vi "Konvolucio MCAN120803 Example Tool.vi"() -> ()   [LabVIEW 2011]
uses:
  <vilib>/Utility/miscctls.llb/LVRowAndColumnUnsignedTypeDef.ctl
  <instrlib>/Konvolucio MCAN120803/Types/CanHandleType.ctl
  <vilib>/Utility/sysdir.llb/System Directory Type.ctl
  <instrlib>/Konvolucio MCAN120803/Types/MessageType.ctl
  <instrlib>/Konvolucio MCAN120803/Public/Attributes/AttrGetRxPendingMsg.vi
  <instrlib>/Konvolucio MCAN120803/Public/Attributes/AttrGetTxPendingMsg.vi
  <instrlib>/Konvolucio MCAN120803/Public/Attributes/AttrGetRxTotal.vi
  <instrlib>/Konvolucio MCAN120803/Public/Attributes/AttrGetTxTotal.vi
  <instrlib>/Konvolucio MCAN120803/Public/Attributes/AttrGetRxErrorCounter.vi
  <instrlib>/Konvolucio MCAN120803/Public/Attributes/AttrGetTxErrorCounter.vi
  <instrlib>/Konvolucio MCAN120803/Public/Attributes/AttrGetRxDrop.vi
  <instrlib>/Konvolucio MCAN120803/Public/Attributes/AttrGetTxDrop.vi
  <instrlib>/Konvolucio MCAN120803/Public/Attributes/AttrSetLoopback.vi
  <instrlib>/Konvolucio MCAN120803/Public/Attributes/AttrSetListenOnly.vi
  <instrlib>/Konvolucio MCAN120803/Public/Attributes/AttrGetAssemblyVersion.vi
  <instrlib>/Konvolucio MCAN120803/Public/Attributes/AttrSetNonAutoRetransmission.vi
  <instrlib>/Konvolucio MCAN120803/Public/Attributes/AttrGetFirmwareRev.vi
  <instrlib>/Konvolucio MCAN120803/Public/Attributes/AttrGetSerialNumber.vi
  <instrlib>/Konvolucio MCAN120803/Public/Attributes/AttrSetTermination.vi
  C:/Program Files/National Instruments/LabVIEW 2011/instr.lib/Konvolucio MCAN120803/Private/Konvolucio.MCAN120803.API.dll
  Private/Konvolucio.MCAN120803.API.dll
  <instrlib>/Konvolucio MCAN120803/Konvolucio MCAN120803.lvlib
panel:
  out "ledStop":bool
  in  "checkBoxListenOnly":bool
  in  "checkBoxNoAutoTx":bool
  in  "checkBoxTermination":bool
  in  "checkBoxLoopback":bool
  in  "Tab 4":enum32{"Incoming messages"}(tab)
  in  "buttonAutoScroll":bool
  in  "buttonSave":bool
  out "Table Control":string[][](table)
  in  "buttonClear":bool
  out "TableRecords":i32
  in  "Tab 3":enum32{"Adapter Info"}(tab)
  out "Serial Number":string
  out "Fw Revision":string
  out "Asm Version":string
  in  "Tab 2":enum32{"Diag"}(tab)
  out "Tx Pending":u32
  out "Rx Pending":u32
  out "Tx Drop":u32
  out "Rx Drop":u32
  out "Tx Error":u32
  out "Rx Error":u32
  out "Tx Total":u32
  out "Rx Total":u32
  in  "Tab":enum32{"Send Simple Message "}(tab)
  in  "buttonSendC":bool
  in  "dataFrameC":string
  in  "lengthC":u8 format="%02x"
  in  "arbIdC":u32 format="%08x"
  in  "buttonSendB":bool
  in  "dataFrameB":string
  in  "lengthB":u8 format="%02x"
  in  "arbIdB":u32 format="%08x"
  in  "dataFrameA":string
  in  "lengthA":u8 format="%02x"
  in  "arbIdA":u32 format="%08x"
  in  "buttonSendA":bool
  in  "comboBaudRate":i32(ring) items=["5.000kBaud", "5.555kBaud", "6.250kBaud", "8.000kBaud", "10.000kBaud", "12.500kBaud", "15.625kBaud", "16.000kBaud", "20.000kBaud", "25.000kBaud", "31.250kBaud", "33.333kBaud", "40.000kBaud", "50.000kBaud", "62.250kBaud", "80.000kBaud", "83.333kBaud", "100.000kBaud", "125.000kBaud", "166.666kBaud", "200.000kBaud", "250.000kBaud", "400.000kBaud", "500.000kBaud", "800.000kBaud", "1.000MBaud"]
  in  "buttonPause":bool
  out "ledOpen":bool
  in  "buttonPlay":bool
  in  "buttonStop":bool
  in  "comboAdapters":i32(ring) items=["CAN Bus Adpater - MCAN120803 3873366E3133 "]
  # "Adapter:"
  # "A"
  # "B"
  # "C"
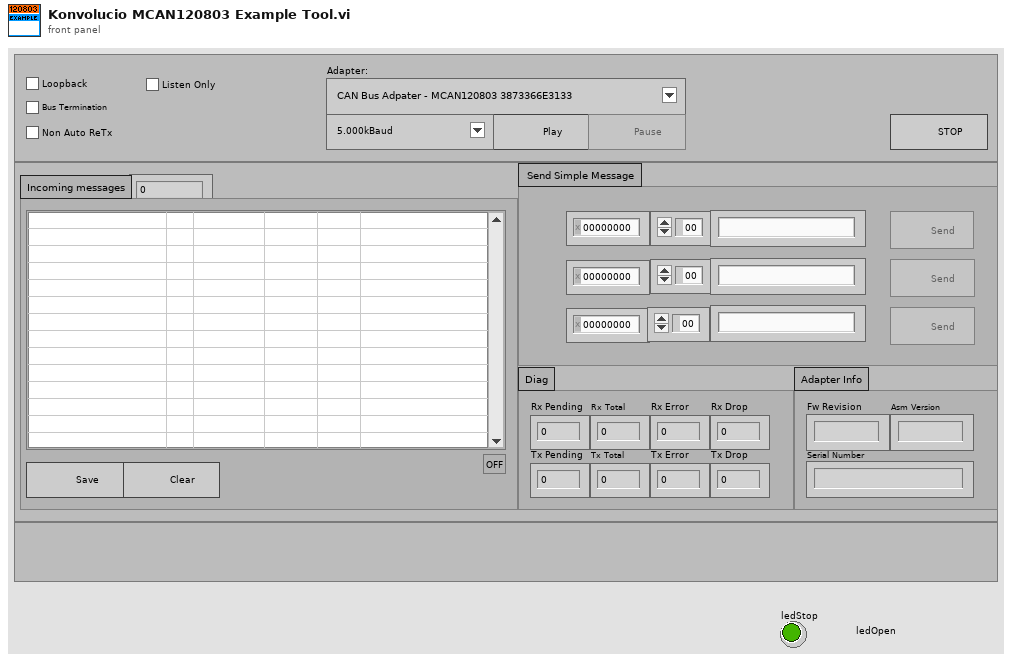
[diagram p1: front panel]
types:
  T1 = enum8{"Enabled", "Disabled", "Disabled and Grayed Out"}
  T2 = typedef "LVRowAndColumnUnsignedTypeDef.ctl" = cluster{"Row":u32, "Column":u32}
  T3 = typedef "Konvolucio MCAN120803.lvlib/BaudRateItemType.ctl" = cluster{"Name":string, "Value":u32}
  T4 = typedef "Konvolucio MCAN120803.lvlib/AdapterItemType.ctl" = cluster{"Name":string, "DeviceDescription":string, "SerialNumber":string, "InUse":bool, "Handle":refnum<k24>}
  T5 = typedef "Konvolucio MCAN120803.lvlib/CanHandleType.ctl" = cluster{"AdapterDevice":refnum<k24>}
  T6 = enum16{"open", "replace", "create", "open or create", "replace or create", "replace or create with confirmation"}
  T7 = typedef "Konvolucio MCAN120803.lvlib/MessageType.ctl" = cluster{"TimeStamp":timestamp, "ArbitrationId":u32, "IsRemote":u8, "DataLength":u8, "Data":u8[]}
  T8 = typedef "System Directory Type.ctl" = i32
  T9 = cluster{"Shift":bool, "Ctrl":bool, "Alt":bool, "Cmd":bool, "Opt":bool}
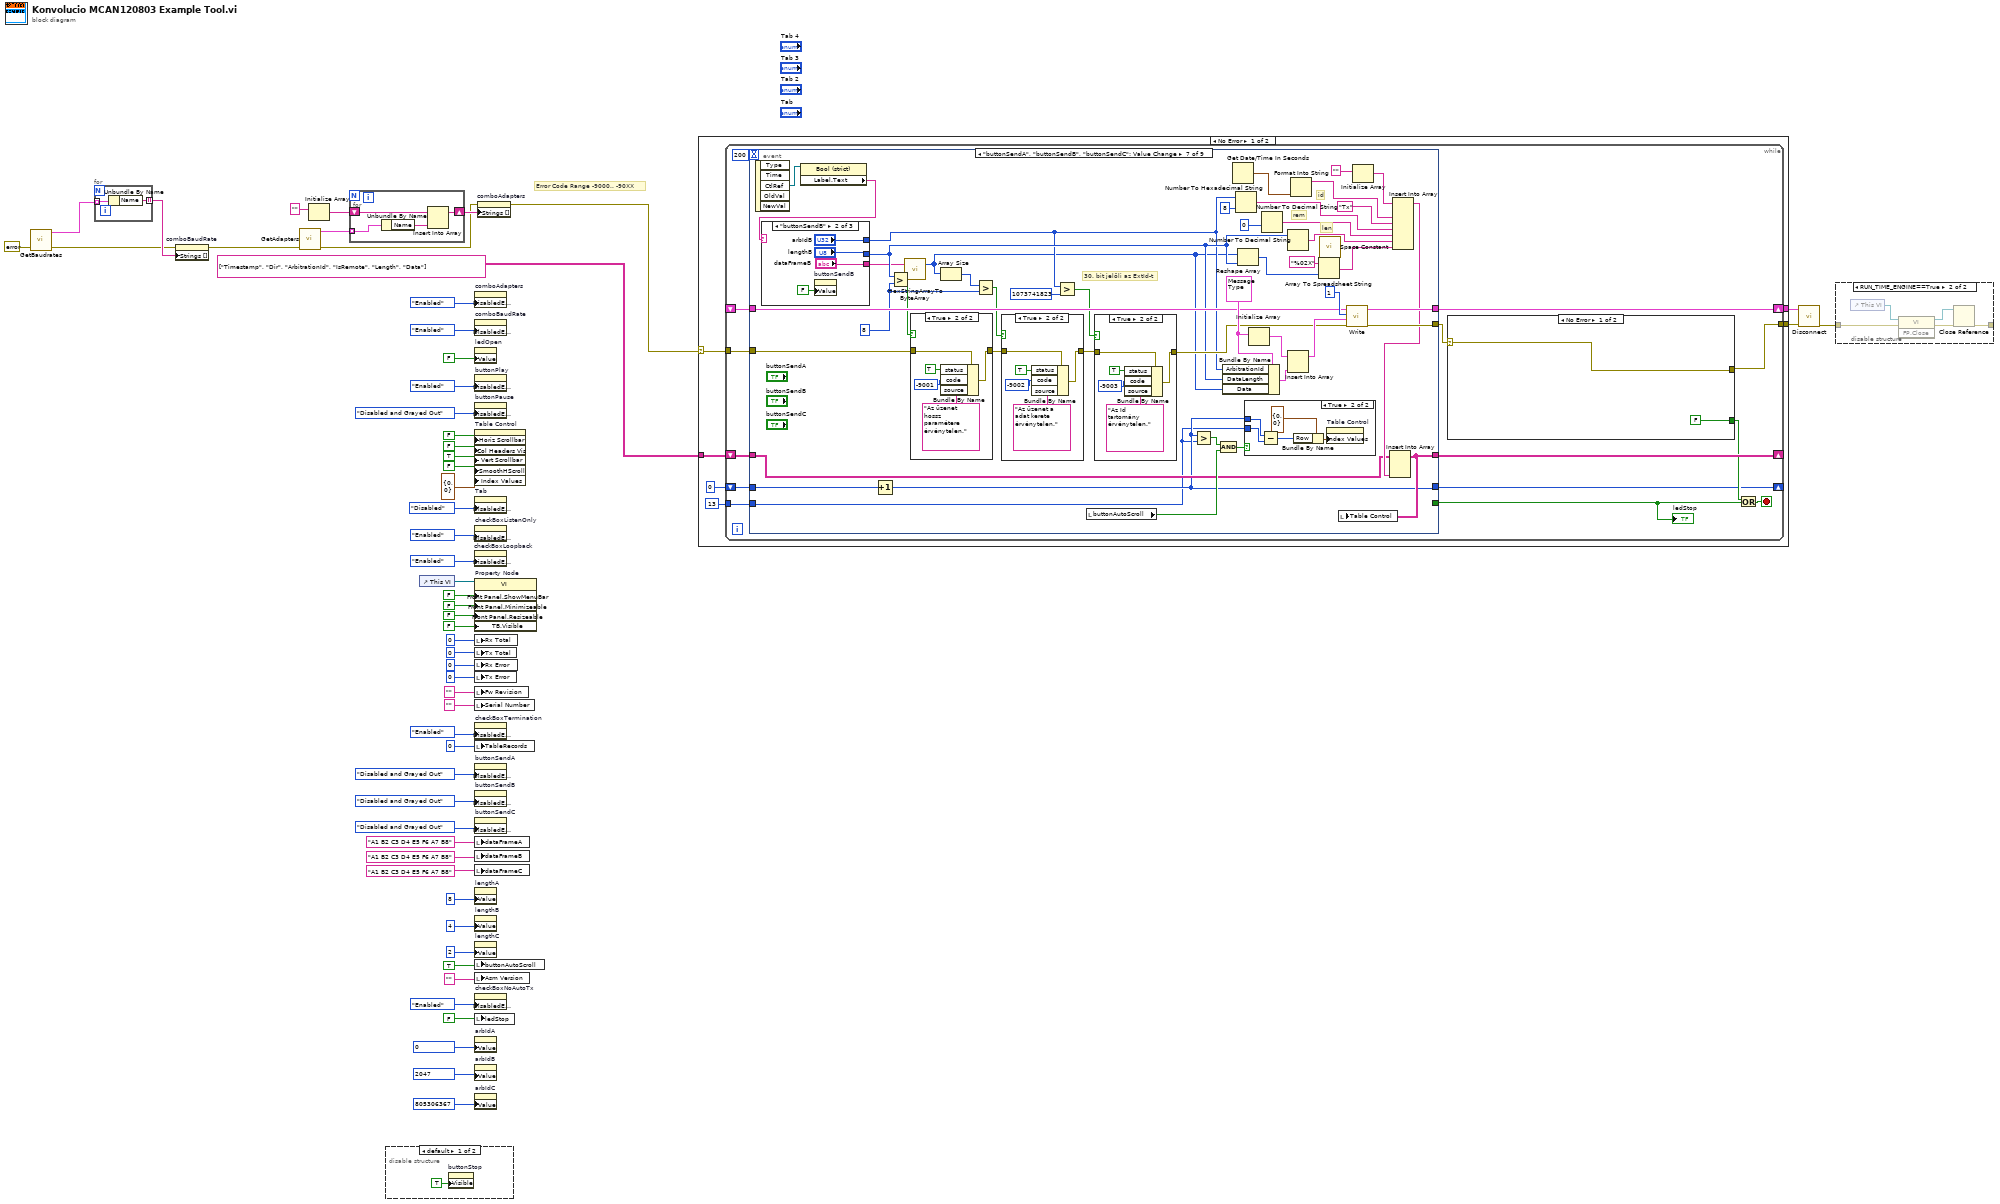
[diagram p0: block diagram]
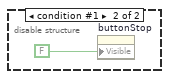
[diagram p2: hidden frame]
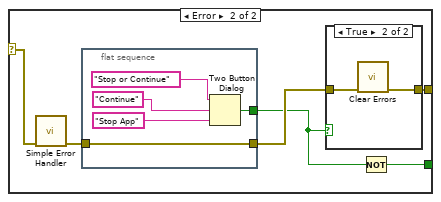
[diagram p4: hidden frame]
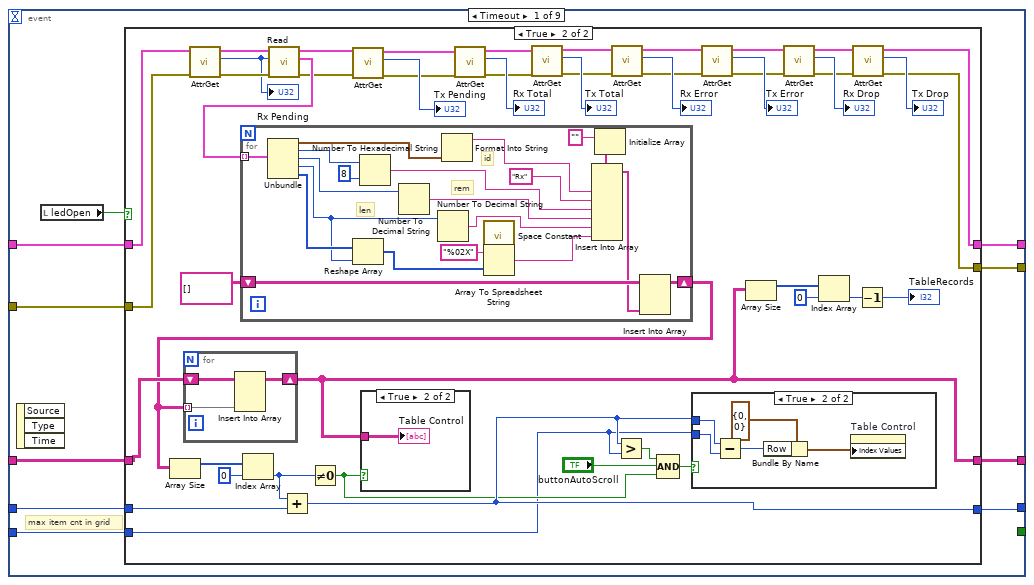
[diagram p6: hidden frame]
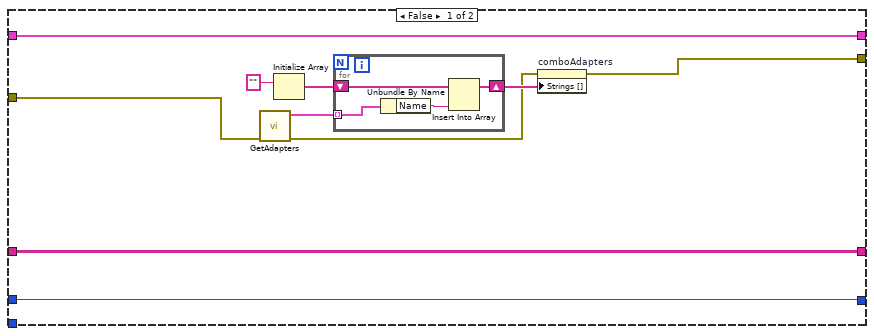
[diagram p7: hidden frame]
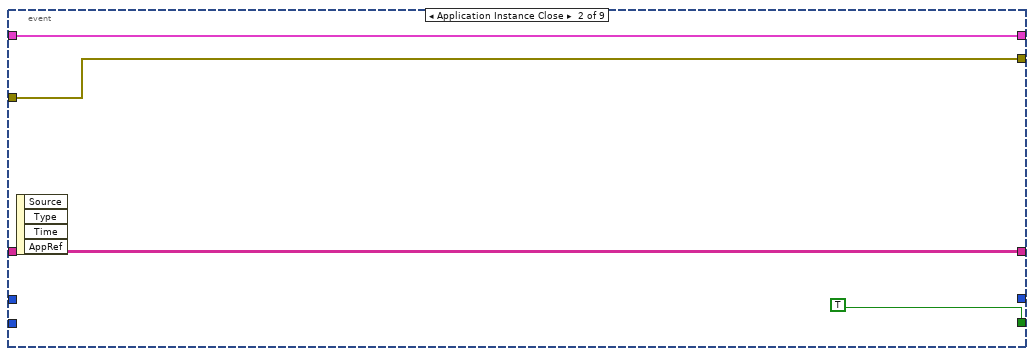
[diagram p10: hidden frame]
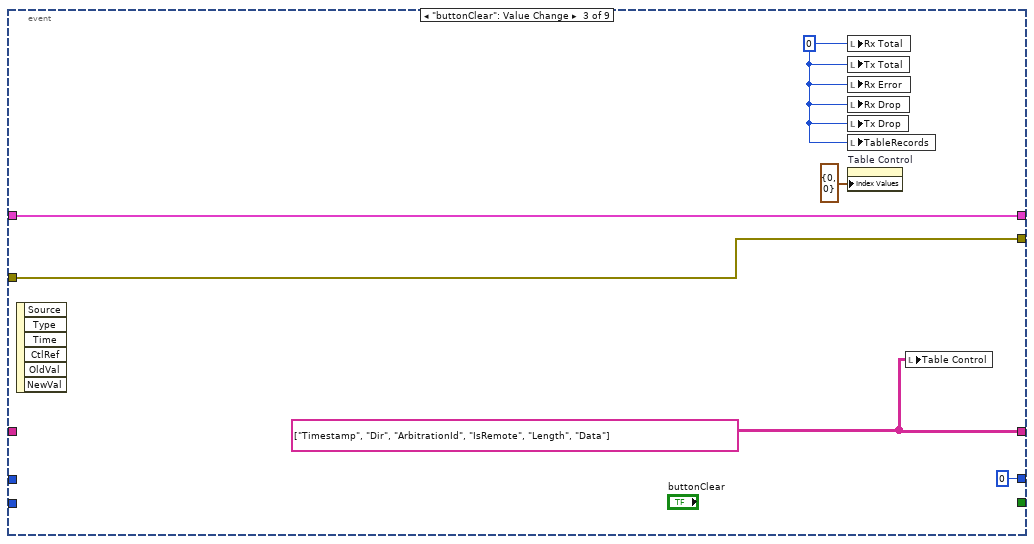
[diagram p11: hidden frame]
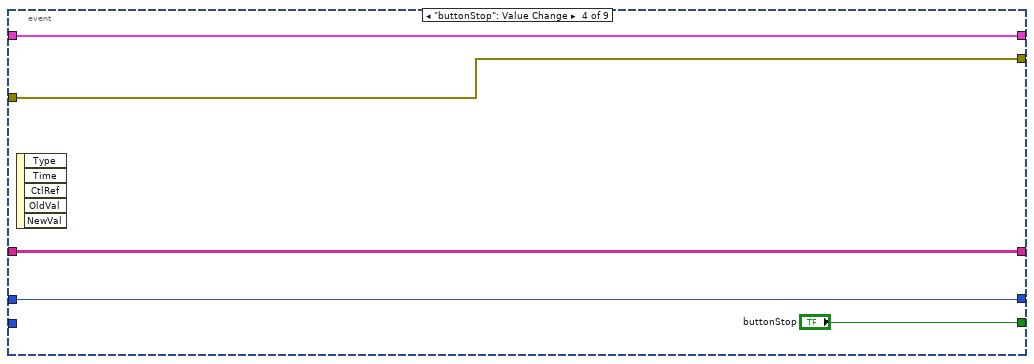
[diagram p12: hidden frame]
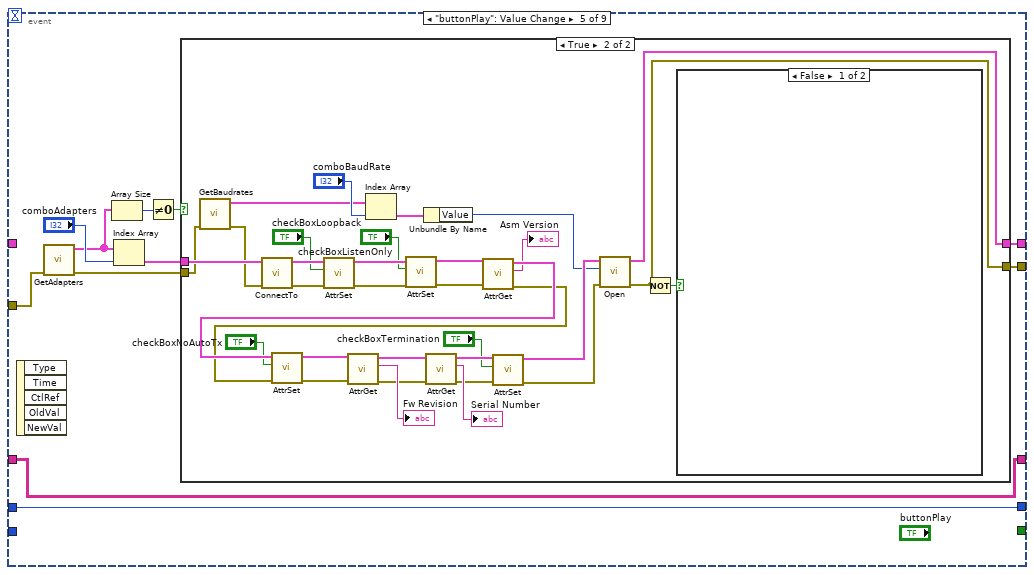
[diagram p13: hidden frame]
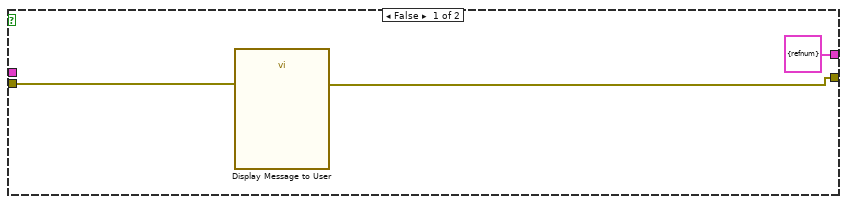
[diagram p14: hidden frame]
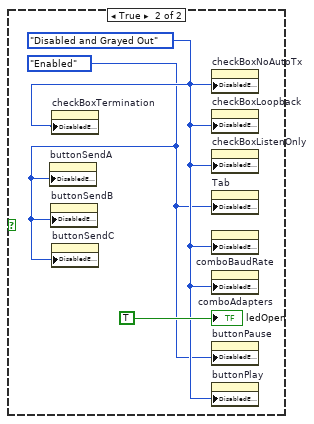
[diagram p15: hidden frame]
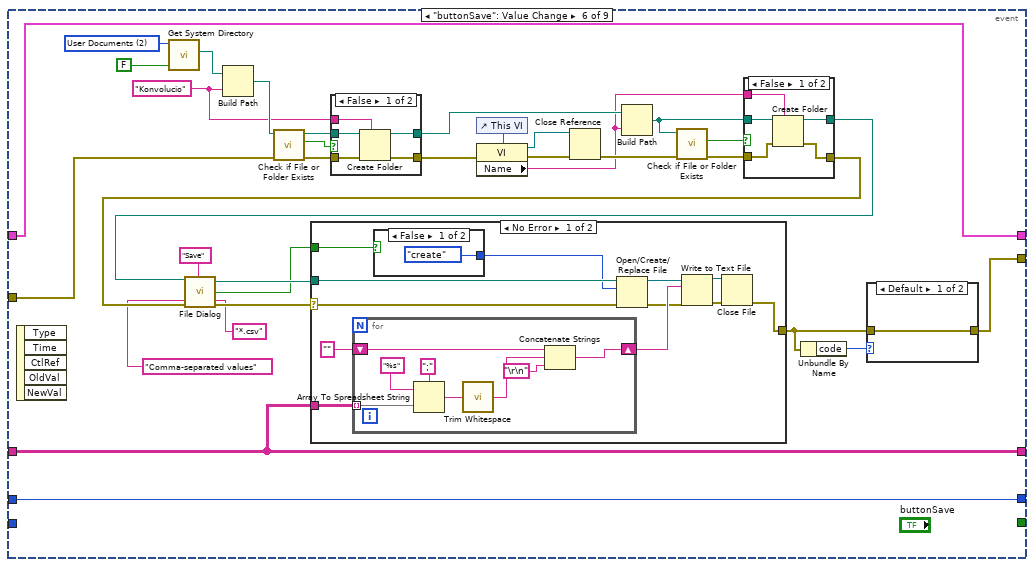
[diagram p16: hidden frame]
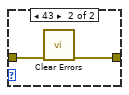
[diagram p17: hidden frame]
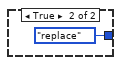
[diagram p18: hidden frame]
diagram:
  # "Error Code Range -9000.. -90XX"
  n1 = call <instrlib>:"GetBaudrates.vi"("error in"=errorcluster {"status"=FALSE, "code"=0, "source"=""}) -> ("error out"=w21:errorcluster, "BaudRateCollection"=w22:T3[])  [unwired: 9 in]
  n2 = for {
    tunnel: w22 -> [w59] mode=indexing
    tunnel: [w58] -> w46 mode=indexing
    n3 = Unbundle By Name(w59) -> ("Name"=w58:string)
  }
  n4 = property on="comboBaudRate" class="Ring (strict)"(error in=w21, "Strings []"=w46) -> (error out=w20:errorcluster)  [unwired: 1 in, 1 out]
  n5 = call <instrlib>:"GetAdapters.vi"("error in"=w20) -> ("error out"=w48:errorcluster, "AdaptersOut"=w57:T4[])  [unwired: 9 in]
  n6 = Initialize Array("") -> (w49:string[])  [unwired: 1 in]
  n7 = for {
    tunnel: w57 -> [w61] mode=indexing
    shift-right: [w62] -> w55
    shift-left: w49 -> [w60]
    n8 = Unbundle By Name(w61) -> ("Name"=w63:string)
    n9 = Insert Into Array(array=w60, new element=w63) -> (w62:string[])  [unwired: 1 in]
  }
  n10 = disable-structure shown="default" {
    frame condition #0 (active) {
      n11 = property on="buttonStop" class="Bool"("Visible"=TRUE) -> ()  [unwired: 2 in, 2 out]
    }
    frame condition #1 {
      n12 = property on="buttonStop" class="Bool"("Visible"=FALSE) -> ()  [unwired: 2 in, 2 out]
    }
  }
  n13 = control-ref of="This VI"() -> (w38:refnum<vi>)
  n14 = property on="comboAdapters" class="Ring (strict)"("DisabledEnum"=T1."Enabled" ("Disabled")) -> ()  [unwired: 2 in, 2 out]
  n15 = property on="comboBaudRate" class="Ring (strict)"("DisabledEnum"=T1."Enabled" ("Disabled")) -> ()  [unwired: 2 in, 2 out]
  n16 = property on="ledOpen" class="Bool (strict)"("Value"=FALSE ("Open")) -> ()  [unwired: 2 in, 2 out]
  n17 = property on="buttonPlay" class="Bool"("DisabledEnum"=T1."Enabled" ("Disabled")) -> ()  [unwired: 2 in, 2 out]
  n18 = property on="buttonPause" class="Bool"("DisabledEnum"=T1."Disabled and Grayed Out" ("Disabled")) -> ()  [unwired: 2 in, 2 out]
  n19 = property on="Table Control" class="Tbl (strict)"("Horiz Scrollbar"=FALSE ("Visible Items:Vertical Scrollbar Visible"), "Col Headers Vis"=FALSE ("Visible Items:Column Headers Visible"), "Vert Scrollbar"=TRUE ("Visible Items:Vertical Scrollbar Visible"), "SmoothHScroll"=FALSE ("Smooth Horizontal Scrolling"), "Index Values"=T2 {"Row"=0, "Column"=0}) -> ()  [unwired: 2 in, 2 out]
  n20 = property on="Tab" class="TabCtl (strict)"("DisabledEnum"=T1."Disabled" ("Disabled")) -> ()  [unwired: 2 in, 2 out]
  n21 = property on="checkBoxListenOnly" class="Bool (strict)"("DisabledEnum"=T1."Enabled" ("Disabled")) -> ()  [unwired: 2 in, 2 out]
  n22 = property on="checkBoxLoopback" class="Bool (strict)"("DisabledEnum"=T1."Enabled" ("Disabled")) -> ()  [unwired: 2 in, 2 out]
  n23 = property on="Property Node" class="VI"(reference=w38, "Front Panel.ShowMenuBar"=FALSE ("Front Panel Window:Show Menu Bar"), "Front Panel.Minimizeable"=FALSE ("Front Panel Window:Minimizable"), "Front Panel.Resizeable"=FALSE ("Front Panel Window:Resizable"), "TB.Visible"=FALSE ("Tool Bar:Visible")) -> ()  [unwired: 1 in, 2 out]
  n24 = local write "Rx Total"(u32 0 ("Total Rx")) -> ()
  n25 = local write "Tx Total"(u32 0 ("Total Tx")) -> ()
  n26 = local write "Rx Error"(u32 0 ("Rx Error Counter")) -> ()
  n27 = local write "Tx Error"(u32 0 ("Tx Error Counter")) -> ()
  n28 = local write "Fw Revision"("" ("Firmware Revision")) -> ()
  n29 = local write "Serial Number"("" ("Serial Number")) -> ()
  n30 = property on="checkBoxTermination" class="Bool (strict)"("DisabledEnum"=T1."Enabled" ("Disabled")) -> ()  [unwired: 2 in, 2 out]
  n31 = local write "TableRecords"(u32 0 ("TableRecords")) -> ()
  n32 = property on="buttonSendA" class="Bool (strict)"("DisabledEnum"=T1."Disabled and Grayed Out" ("Disabled")) -> ()  [unwired: 2 in, 2 out]
  n33 = property on="buttonSendB" class="Bool (strict)"("DisabledEnum"=T1."Disabled and Grayed Out" ("Disabled")) -> ()  [unwired: 2 in, 2 out]
  n34 = property on="buttonSendC" class="Bool (strict)"("DisabledEnum"=T1."Disabled and Grayed Out" ("Disabled")) -> ()  [unwired: 2 in, 2 out]
  n35 = local write "dataFrameA"("A1 B2 C3 D4 E5 F6 A7 B8" ("dataFrame1")) -> ()
  n36 = local write "dataFrameB"("A1 B2 C3 D4 E5 F6 A7 B8" ("dataFrameB")) -> ()
  n37 = local write "dataFrameC"("A1 B2 C3 D4 E5 F6 A7 B8" ("dataFrameB")) -> ()
  n38 = property on="lengthA" class="DigNum (strict)"("Value"=u8 8 ("lengthA")) -> ()  [unwired: 2 in, 2 out]
  n39 = property on="lengthB" class="DigNum (strict)"("Value"=u8 4 ("lengthB")) -> ()  [unwired: 2 in, 2 out]
  n40 = property on="lengthC" class="DigNum (strict)"("Value"=u8 2 ("lengthC")) -> ()  [unwired: 2 in, 2 out]
  n41 = local write "buttonAutoScroll"(TRUE ("buttonAutoScroll")) -> ()
  n42 = local write "Asm Version"("" ("Asm Version")) -> ()
  n43 = property on="checkBoxNoAutoTx" class="Bool (strict)"("DisabledEnum"=T1."Enabled" ("Disabled")) -> ()  [unwired: 2 in, 2 out]
  n44 = local write "ledStop"(FALSE ("ledStop")) -> ()
  n45 = property on="arbIdA" class="DigNum (strict)"("Value"=u32 0 ("arbIdA")) -> ()  [unwired: 2 in, 2 out]
  n46 = property on="arbIdB" class="DigNum (strict)"("Value"=u32 2047 ("arbIdA")) -> ()  [unwired: 2 in, 2 out]
  n47 = property on="arbIdC" class="DigNum (strict)"("Value"=u32 805306367 ("arbIdA")) -> ()  [unwired: 2 in, 2 out]
  n48 = property on="comboAdapters" class="Ring (strict)"(error in=w48, "Strings []"=w55) -> (error out=w47:errorcluster)  [unwired: 1 in, 1 out]
  n49 = case shown="No Error" w47 {
    selector: w47 -> [w71 w450]
    tunnel: [w70 w450] -> w19
    tunnel: [w69 T5 {"AdapterDevice"=refnum} ("HandleOut")] -> w54
    tunnel: string[][] [["Timestamp", "Dir", "ArbitrationId", "IsRemote", "Length", "Data"]] ("Table Control 3") -> [w68 _]
    frame No Error {
      n50 = while {
        tunnel: w71 -> [w85]
        tunnel: [w75] -> w70
        shift-right: [w84] -> w69
        shift-left: _ -> [w83]
        shift-right: [w80] -> _
        shift-left: w68 -> [w81]
        shift-right: [w74] -> _
        shift-left: 0 ("x-1") -> [w73]
        tunnel: 13 ("y") -> [w72]
        stop <- w79 stop-if-true
        n51 = event shown="[6] \"buttonSendA\", \"buttonSendB\", \"buttonSendC\": Value Change" {
          selector: _ -> [_ _ _ _ _ _ _ _ _]
          dyn-events: _ -> [_ _ _ _ _ _ _ _ _]
          timeout: 200 -> [_ _ _ _ _ _ _ _ _]
          tunnel: [_ TRUE ("buttonStop") _ "buttonStop" _ _ _ _ _] -> w76
          tunnel: w85 -> [w110 w204 w211 w214 w223 w286 w359 w428 w446]
          tunnel: [w109 w204 w211 w214 w225 w269 w383 w428 w447] -> w78
          tunnel: [w108 w205 w212 w216 w226 w272 w381 w427 w444] -> w84
          tunnel: w83 -> [w111 w205 w212 w216 _ w272 w380 w427 w444]
          tunnel: w81 -> [w107 w203 _ w215 w218 w280 w358 w430 w437]
          tunnel: [w105 w203 w209 w215 w218 w280 w360 w430 w437] -> w80
          tunnel: [w103 _ 0 ("Total Rx") w213 w219 w268 w353 w429 w440] -> w74
          tunnel: w73 -> [w104 _ _ w213 w219 w268 w364 w429 w440]
          tunnel: w72 -> [w102 _ _ _ _ _ w352 _ _]
          event Timeout {
            # "max item cnt in grid"
            n52 = event-data() -> ()  [unwired: 1 in, 3 out]
            n53 = local read "ledOpen"() -> (w106:bool)
            n54 = case shown="True" w106 {
              tunnel: w111 -> [w121 w169]
              tunnel: w110 -> [w115 w170]
              tunnel: [w113 w150] -> w109
              tunnel: [w121 w149] -> w108
              tunnel: w107 -> [w120 w143]
              tunnel: [w120 w144] -> w105
              tunnel: w104 -> [w112 w140]
              tunnel: [w112 w139] -> w103
              tunnel: w102 -> [_ w132]
              frame False {
                n55 = call <instrlib>:"GetAdapters.vi"("error in"=w115) -> ("error out"=w114:errorcluster, "AdaptersOut"=w116:T4[])  [unwired: 9 in]
                n56 = Initialize Array("") -> (w118:string[])  [unwired: 1 in]
                n57 = for {
                  tunnel: w116 -> [w123] mode=indexing
                  shift-right: [w124] -> w119
                  shift-left: w118 -> [w122]
                  n58 = Unbundle By Name(w123) -> ("Name"=w125:string)
                  n59 = Insert Into Array(array=w122, new element=w125) -> (w124:string[])  [unwired: 1 in]
                }
                n60 = property on="comboAdapters" class="Ring (strict)"(error in=w114, "Strings []"=w119) -> (error out=w113:errorcluster)  [unwired: 1 in, 1 out]
              }
              frame True {
                n61 = call-poly <instrlib>:"AttrGet.vi"("error in"=w170, "CanHandleIn"=w169) -> ("error out"=w171:errorcluster, "Value"=w131:i32, "CanHandleOut"=w172:T5)  [unwired: 7 in]
                "Rx Pending" <- w131
                n62 = call <instrlib>:"Read.vi"("error in"=w171, "Request Number of Message"=w131, "CanHandleIn"=w172) -> ("error out"=w130:errorcluster, "Messages"=w167:T7[], "CanHandleOut"=w129:T5)  [unwired: 6 in]
                n63 = for {
                  tunnel: w167 -> [w199] mode=indexing
                  shift-right: [w189] -> w138
                  shift-left: string[][] [] -> [w190]
                  # "len"
                  # "rem"
                  # "id"
                  n64 = Unbundle(w199) -> ("TimeStamp"=w187:timestamp, "ArbitrationId"=w194:u32, "IsRemote"=w195:u8, "DataLength"=w185:u8, "Data"=w196:u8[])
                  n65 = Reshape Array(w196, w185) -> (w186:u8[])
                  n66 = Number To Hexadecimal String(1:i16 8 ("width (-)"), 2:w194) -> (0:w181:string)
                  n67 = Number To Decimal String(number=w195) -> (decimal integer string=w182:string)  [unwired: 1 in]
                  n68 = Number To Decimal String(number=w185) -> (decimal integer string=w183:string)  [unwired: 1 in]
                  n69 = Format Into String(w187) -> (resulting string=w180:string)  [unwired: 3 in, 1 out]
                  n70 = call <vilib>:"Space Constant.vi"() -> ("String"=w197:string)
                  n71 = Array To Spreadsheet String(delimiter (Tab)=w197, array=w186, 3:"%02X" ("format string")) -> (spreadsheet string=w184:string)
                  n72 = Initialize Array("") -> (w192:string[])  [unwired: 1 in]
                  n73 = Insert Into Array(array=w192, new element #1=w180, new element #2="Rx" ("new element/subarray"), new element #3=w181, new element #4=w182, new element #5=w183, new element #6=w184) -> (w188:string[])  [unwired: 1 in]
                  n74 = Insert Into Array(array=w190, new element=w188) -> (w189:string[][])  [unwired: 2 in]
                }
                n75 = Array Size(array=w138) -> (size(s)=w142:i32[])
                n76 = for {
                  shift-right: [w202] -> w144
                  shift-left: w143 -> [w201]
                  tunnel: w138 -> [w200] mode=indexing
                  n77 = Insert Into Array(array=w201, new element=w200) -> (w202:string[][])  [unwired: 2 in]
                }
                n78 = Index Array(array=w142, index=0) -> (element=w137:i32)
                n79 = Add(x=w137, y=w140) -> (x+y=w139:i32)
                n80 = Not Equal To 0?(x=w137) -> (x != 0?=w134:bool)
                n81 = call-poly <instrlib>:"AttrGet.vi"("error in"=w130, "CanHandleIn"=w129) -> ("error out"=w127:errorcluster, "Value"=→"Tx Pending":u32, "CanHandleOut"=w126:T5)  [unwired: 7 in]
                n82 = case shown="True" w134 {
                  tunnel: w144 -> [_ w173]
                  frame False {
                  }
                  frame True {
                    "Table Control" <- w173
                  }
                }
                n83 = call-poly <instrlib>:"AttrGet.vi"("error in"=w127, "CanHandleIn"=w126) -> ("error out"=w164:errorcluster, "Value"=→"Rx Total":u32, "CanHandleOut"=w165:T5)  [unwired: 7 in]
                n84 = call-poly <instrlib>:"AttrGet.vi"("error in"=w164, "CanHandleIn"=w165) -> ("error out"=w161:errorcluster, "Value"=→"Tx Total":u32, "CanHandleOut"=w162:T5)  [unwired: 7 in]
                n85 = call-poly <instrlib>:"AttrGet.vi"("error in"=w161, "CanHandleIn"=w162) -> ("error out"=w158:errorcluster, "Value"=→"Rx Error":u32, "CanHandleOut"=w159:T5)  [unwired: 7 in]
                n86 = Greater?(x=w139, y=w132) -> (0:w136:bool)
                n87 = Compound Arithmetic op=AND(w136, "buttonAutoScroll", w134) -> (w133:bool)
                n88 = case shown="True" w133 {
                  tunnel: w132 -> [_ w175]
                  tunnel: w139 -> [_ w176]
                  frame False {
                  }
                  frame True {
                    n89 = Subtract(x=w176, y=w175) -> (x-y=w177:i32)
                    n90 = Bundle By Name(cluster=T2 {"Row"=0, "Column"=0} ("Index Values"), "Row"=w177) -> (w174:T2)
                    n91 = property on="Table Control" class="Tbl (strict)"("Index Values"=w174) -> ()  [unwired: 2 in, 2 out]
                  }
                }
                n92 = call-poly <instrlib>:"AttrGet.vi"("error in"=w158, "CanHandleIn"=w159) -> ("error out"=w156:errorcluster, "Value"=→"Tx Error":u32, "CanHandleOut"=w155:T5)  [unwired: 7 in]
                n93 = Array Size(array=w144) -> (size(s)=w148:i32[])
                n94 = call-poly <instrlib>:"AttrGet.vi"("error in"=w156, "CanHandleIn"=w155) -> ("error out"=w153:errorcluster, "Value"=→"Rx Drop":u32, "CanHandleOut"=w152:T5)  [unwired: 7 in]
                n95 = Index Array(array=w148, index=0) -> (element=w146:i32)
                n96 = call-poly <instrlib>:"AttrGet.vi"("error in"=w153, "CanHandleIn"=w152) -> ("error out"=w150:errorcluster, "Value"=→"Tx Drop":u32, "CanHandleOut"=w149:T5)  [unwired: 7 in]
                n97 = Decrement(x=w146) -> (x-1=→"TableRecords":i32)
              }
            }
          }
          event Application Instance Close {
            n98 = event-data() -> ()  [unwired: 1 in, 4 out]
          }
          event "buttonClear": Value Change {
            w208 = u32 0 ("Total Rx")
            w209 = string[][] [["Timestamp", "Dir", "ArbitrationId", "IsRemote", "Length", "Data"]] ("Table Control 3")
            n99 = event-data() -> ()  [unwired: 1 in, 6 out]
            n100 = local write "Rx Total"(w208) -> ()
            n101 = local write "Tx Total"(w208) -> ()
            n102 = local write "Rx Error"(w208) -> ()
            n103 = local write "Rx Drop"(w208) -> ()
            n104 = local write "Tx Drop"(w208) -> ()
            n105 = local write "TableRecords"(w208) -> ()
            n106 = property on="Table Control" class="Tbl (strict)"("Index Values"=T2 {"Row"=0, "Column"=0}) -> ()  [unwired: 2 in, 2 out]
            n107 = local write "Table Control"(w209) -> ()
          }
          event "buttonStop": Value Change {
            n108 = event-data() -> ()  [unwired: 1 in, 5 out]
          }
          event "buttonPlay": Value Change {
            n109 = event-data() -> ()  [unwired: 1 in, 5 out]
            n110 = call <instrlib>:"GetAdapters.vi"("error in"=w223) -> ("error out"=w224:errorcluster, "AdaptersOut"=w222:T4[])  [unwired: 9 in]
            n111 = Array Size(array=w222) -> (size(s)=w220:i32)
            n112 = Index Array(array=w222, index="comboAdapters") -> (element=w227:T4)
            n113 = Not Equal To 0?(x=w220) -> (x != 0?=w221:bool)
            n114 = case shown="True" w221 {
              tunnel: w227 -> [_ w264]
              tunnel: [T5 {"AdapterDevice"=refnum} ("MCanHandleOut") w260] -> w226
              tunnel: [w229 w259] -> w225
              tunnel: w224 -> [w230 w243]
              frame False {
                n115 = call "Display Message to User"("error in (no error)"=w230) -> ("error out"=w229:errorcluster)  [unwired: 9 in, 1 out]
              }
              frame True {
                n116 = call <instrlib>:"GetBaudrates.vi"("error in"=w243) -> ("error out"=w242:errorcluster, "BaudRateCollection"=w241:T3[])  [unwired: 9 in]
                n117 = call <instrlib>:"ConnectTo.vi"("error in"=w242, "AdapterIn"=w264) -> ("error out"=w258:errorcluster, "CanHandleOut"=w257:T5)  [unwired: 8 in]
                n118 = call-poly <instrlib>:"AttrSet.vi"("error in"=w258, "Enabled"="checkBoxLoopback", "CanHandleIn"=w257) -> ("error out"=w256:errorcluster, "CanHandleOut"=w255:T5)  [unwired: 6 in]
                n119 = Index Array(array=w241, index="comboBaudRate") -> (element=w261:T3)
                n120 = call-poly <instrlib>:"AttrSet.vi"("error in"=w256, "Enabled"="checkBoxListenOnly", "CanHandleIn"=w255) -> ("error out"=w240:errorcluster, "CanHandleOut"=w239:T5)  [unwired: 6 in]
                n121 = Unbundle By Name(w261) -> ("Value"=w244:u32)
                n122 = call-poly <instrlib>:"AttrGet.vi"("error in"=w240, "MCanHandleIn"=w239) -> ("error out"=w237:errorcluster, "Value"=→"Asm Version":string, "MCanHandleOut"=w238:T5)  [unwired: 7 in]
                n123 = call-poly <instrlib>:"AttrSet.vi"("error in"=w237, "Enabled"="checkBoxNoAutoTx", "CanHandleIn"=w238) -> ("error out"=w253:errorcluster, "CanHandleOut"=w254:T5)  [unwired: 6 in]
                n124 = call-poly <instrlib>:"AttrGet.vi"("error in"=w253, "CanHandleIn"=w254) -> ("error out"=w250:errorcluster, "Value"=→"Fw Revision":string, "CanHandleOut"=w251:T5)  [unwired: 7 in]
                n125 = call-poly <instrlib>:"AttrGet.vi"("error in"=w250, "CanHandleIn"=w251) -> ("error out"=w247:errorcluster, "Value"=→"Serial Number":string, "CanHandleOut"=w248:T5)  [unwired: 7 in]
                n126 = call-poly <instrlib>:"AttrSet.vi"("error in"=w247, "Enabled"="checkBoxTermination", "CanHandleIn"=w248) -> ("error out"=w245:errorcluster, "CanHandleOut"=w246:T5)  [unwired: 6 in]
                n127 = call <instrlib>:"Open.vi"("error in"=w245, "Baudrate"=w244, "CanHandleIn"=w246) -> ("error out"=w259:errorcluster, "CanHandleOut"=w260:T5)  [unwired: 7 in]
                n128 = Not(x=w259) -> (.not. x?=w263:bool)
                n129 = case shown="False" w263 {
                  frame False {
                  }
                  frame True {
                    w266 = T1."Disabled and Grayed Out" ("Disabled")
                    w265 = T1."Enabled" ("Disabled")
                    n130 = property on="buttonSendA" class="Bool (strict)"("DisabledEnum"=w265) -> ()  [unwired: 2 in, 2 out]
                    n131 = property on="buttonSendB" class="Bool (strict)"("DisabledEnum"=w265) -> ()  [unwired: 2 in, 2 out]
                    n132 = property on="checkBoxTermination" class="Bool (strict)"("DisabledEnum"=w266) -> ()  [unwired: 2 in, 2 out]
                    n133 = property on="buttonSendC" class="Bool (strict)"("DisabledEnum"=w265) -> ()  [unwired: 2 in, 2 out]
                    n134 = property on="checkBoxNoAutoTx" class="Bool (strict)"("DisabledEnum"=w266) -> ()  [unwired: 2 in, 2 out]
                    n135 = property on="checkBoxLoopback" class="Bool (strict)"("DisabledEnum"=w266) -> ()  [unwired: 2 in, 2 out]
                    n136 = property on="checkBoxListenOnly" class="Bool (strict)"("DisabledEnum"=w266) -> ()  [unwired: 2 in, 2 out]
                    n137 = property on="Tab" class="TabCtl (strict)"("DisabledEnum"=w265) -> ()  [unwired: 2 in, 2 out]
                    n138 = property on="comboBaudRate" class="Ring (strict)"("DisabledEnum"=w266) -> ()  [unwired: 2 in, 2 out]
                    n139 = property on="comboAdapters" class="Ring (strict)"("DisabledEnum"=w266) -> ()  [unwired: 2 in, 2 out]
                    n140 = property on="buttonPause" class="Bool"("DisabledEnum"=w265) -> ()  [unwired: 2 in, 2 out]
                    n141 = property on="buttonPlay" class="Bool"("DisabledEnum"=w266) -> ()  [unwired: 2 in, 2 out]
                    "ledOpen" <- TRUE ("Open")
                  }
                }
              }
            }
          }
          event "buttonSave": Value Change {
            w290 = "Konvolucio" ("prompt (Create Folder)")
            w300 = T8 2 items=["User Home"=0, "User Desktop"=1, "User Documents"=2, "User Application Data"=3, "User Preferences"=4, "User Temporary"=5, "Public Documents"=6, "Public Application Data"=7, "Public Preferences"=8, "Public Cache"=13, "System Core Libraries"=9, "System Installed Libraries"=10, "Application Files"=11, "Boot Volume Root"=12] ("system directory type")
            n142 = event-data() -> ()  [unwired: 1 in, 5 out]
            n143 = call <vilib>:"Get System Directory.vi"("create directory if not found? (F)"=FALSE, "system directory type"=w300) -> ("system directory"=w295:path)  [unwired: 9 in]
            n144 = Build Path(base path=w295, name or relative path=w290) -> (appended path=w294:path)
            n145 = call <vilib>:"Check if File or Folder Exists.vi"("error in (no error)"=w286, "path"=w294) -> ("error out"=w292:errorcluster, "file or folder exists?"=w293:bool, "dup path"=w291:path)  [unwired: 7 in]
            n146 = case shown="False" w293 {
              tunnel: [w338 w340] -> w289
              tunnel: w292 -> [w337 w340]
              tunnel: w291 -> [w336 w339]
              tunnel: w290 -> [w335 _]
              tunnel: [w334 w339] -> w288
              frame False {
                n147 = Create Folder(prompt (Create Folder)=w335, path (use dialog)=w336, error in=w337) -> (created path=w334:path, error out=w338:errorcluster)  [unwired: 1 out]
              }
              frame True {
              }
            }
            n148 = control-ref of="This VI"() -> (w298:refnum<vi>)
            n149 = property class="VI"(reference=w298, error in=w289) -> (reference out=w296:refnum<vi>, error out=w297:errorcluster, "Name"=w282:string)
            n150 = Close Reference(reference=w296, error in (no error)=w297) -> (error out=w287:errorcluster)
            n151 = Build Path(base path=w288, name or relative path=w282) -> (appended path=w284:path)
            n152 = call <vilib>:"Check if File or Folder Exists.vi"("error in (no error)"=w287, "path"=w284) -> ("error out"=w283:errorcluster, "file or folder exists?"=w285:bool)  [unwired: 7 in, 1 out]
            n153 = case shown="False" w285 {
              tunnel: [w331 w332] -> w281
              tunnel: [w330 w333] -> w279
              tunnel: w284 -> [w329 w333]
              tunnel: w283 -> [w328 w332]
              tunnel: w282 -> [w327 _]
              frame False {
                n154 = Create Folder(prompt (Create Folder)=w327, path (use dialog)=w329, error in=w328) -> (created path=w330:path, error out=w331:errorcluster)  [unwired: 1 out]
              }
              frame True {
              }
            }
            n155 = call "File Dialog"("start path"=w279, "button label"="Save", "error in"=w281, "pattern (all files)"="*.csv", "pattern label"="Comma-separated values") -> ("selected path"=w277:path, "exists"=w274:bool, "error out"=w276:errorcluster)  [unwired: 7 in, 1 out]
            n156 = case shown="No Error" w276 {
              selector: w276 -> [w305 w326]
              tunnel: w280 -> [w315 _]
              tunnel: [w310 w326] -> w270
              tunnel: w277 -> [w307 _]
              tunnel: w274 -> [w304 _]
              frame No Error {
                n157 = for {
                  tunnel: w315 -> [w323] mode=indexing
                  shift-right: [w319] -> w313
                  shift-left: "" -> [w321]
                  n158 = Array To Spreadsheet String(delimiter (Tab)=";", array=w323, 3:"%s" ("format string")) -> (spreadsheet string=w325:string)
                  n159 = call <vilib>:"Trim Whitespace.vi"("string"=w325) -> ("trimmed string"=w320:string)  [unwired: 1 in]
                  n160 = Concatenate Strings(w321, w320, "\r\n") -> (w319:string)
                }
                n161 = case shown="False" w304 {
                  tunnel: [T6."create" ("operation (0:open)") T6."replace" ("operation (0:open)")] -> w306
                  frame False {
                  }
                  frame True {
                  }
                }
                n162 = Open/Create/Replace File(file path (use dialog)=w307, error in=w305, operation (0:open)=w306) -> (refnum out=w308:refnum<file>, error out=w309:errorcluster)  [unwired: 3 in, 1 out]
                n163 = Write to Text File(file (use dialog)=w308, text=w313, error in=w309) -> (refnum out=w311:refnum<file>, error out=w312:errorcluster)  [unwired: 1 in, 1 out]
                n164 = Close File(refnum=w311, error in=w312) -> (error out=w310:errorcluster)  [unwired: 1 out]
              }
              frame Error {
              }
            }
            n165 = Unbundle By Name(w270) -> ("code"=w271:i32)
            n166 = case shown="Default" w271 {
              tunnel: w270 -> [w301 w303]
              tunnel: [w301 w302] -> w269
              frame Default {
              }
              frame 43 {
                n167 = call <vilib>:"Clear Errors.vi"("error in (no error)"=w303) -> ("error out"=w302:errorcluster)  [unwired: 6 in]
              }
            }
          }
          event "buttonSendA", "buttonSendB", "buttonSendC": Value Change {
            w347 = u8 8 ("lengthA")
            w384 = T7 {"TimeStamp"=timestamp(0 s since 1904-01-01), "ArbitrationId"=0, "IsRemote"=0, "DataLength"=0, "Data"=[]}
            # "30. bit jelöli az ExtId-t"
            # "len"
            # "id"
            # "rem"
            n168 = event-data() -> ("CtlRef"=w346:refnum<vi>)  [unwired: 1 in, 4 out]
            n169 = property class="Bool (strict)"(reference=w346) -> ("Label.Text"=w344:string)  [unwired: 1 in, 2 out]
            n170 = case shown="\"buttonSendB\"" w344 {
              tunnel: ["arbIdA" "arbIdB" "arbIdC"] -> w342
              tunnel: ["lengthA" "lengthB" "lengthC"] -> w345
              tunnel: ["dataFrameA" "dataFrameB" "dataFrameC"] -> w343
              frame "buttonSendA", Default {
                n171 = property on="buttonSendA" class="Bool (strict)"("Value"=FALSE ("buttonSendA")) -> ()  [unwired: 2 in, 2 out]
              }
              frame "buttonSendB" {
                n172 = property on="buttonSendB" class="Bool (strict)"("Value"=FALSE ("buttonSendB")) -> ()  [unwired: 2 in, 2 out]
              }
              frame "buttonSendC" {
                n173 = property on="buttonSendC" class="Bool (strict)"("Value"=FALSE ("buttonSendC")) -> ()  [unwired: 2 in, 2 out]
              }
            }
            n174 = Increment(x=w364) -> (x+1=w353:i32)
            n175 = Greater?(x=w345, y=w347) -> (0:w357:bool)
            n176 = call <instrlib>:"HexStringArrayToByteArray.vi"("HexStirngArray"=w343) -> ("ByteArrayOut"=w341:u8[])  [unwired: 2 in]
            n177 = case shown="True" w357 {
              tunnel: w359 -> [w412 w417]
              tunnel: [w412 w416] -> w354
              frame False {
              }
              frame True {
                n178 = Bundle By Name(cluster=w417, "status"=TRUE, "code"=-9001, "source"="Az üzenet hossz paramétere érvénytelen.") -> (w416:errorcluster)
              }
            }
            n179 = Array Size(array=w341) -> (size(s)=w355:i32)
            n180 = Greater?(x=w355, y=w347) -> (0:w356:bool)
            n181 = case shown="True" w356 {
              tunnel: w354 -> [w406 w411]
              tunnel: [w406 w410] -> w351
              frame False {
              }
              frame True {
                n182 = Bundle By Name(cluster=w411, "status"=TRUE, "code"=-9002, "source"="Az üzenet a adat kerete érvénytelen.") -> (w410:errorcluster)
              }
            }
            n183 = Greater?(x=w342, y=u32 1073741823 ("arbIdA")) -> (0:w349:bool)
            n184 = local read "buttonAutoScroll"() -> (w361:bool)
            n185 = case shown="True" w349 {
              tunnel: w351 -> [w400 w405]
              tunnel: [w400 w404] -> w350
              frame False {
              }
              frame True {
                n186 = Bundle By Name(cluster=w405, "status"=TRUE, "code"=-9003, "source"="Az Id tartomány érvénytelen.") -> (w404:errorcluster)
              }
            }
            n187 = Greater?(x=w353, y=w352) -> (0:w362:bool)
            n188 = Compound Arithmetic op=AND(w362, w361) -> (w363:bool)
            n189 = Bundle By Name(cluster=w384, "ArbitrationId"=w342, "DataLength"=w345, "Data"=w341) -> (w385:T7)
            n190 = Get Date/Time In Seconds() -> (seconds since 1Jan1904=w372:timestamp)
            n191 = Number To Hexadecimal String(1:i16 8 ("width (-)"), 2:w342) -> (0:w378:string)
            n192 = Reshape Array(w341, w345) -> (w369:u8[])
            n193 = case shown="True" w363 {
              tunnel: w352 -> [_ w419]
              tunnel: w353 -> [_ w420]
              frame False {
              }
              frame True {
                n194 = Subtract(x=w420, y=w419) -> (x-y=w421:i32)
                n195 = Bundle By Name(cluster=T2 {"Row"=0, "Column"=0} ("Index Values"), "Row"=w421) -> (w418:T2)
                n196 = property on="Table Control" class="Tbl (strict)"("Index Values"=w418) -> ()  [unwired: 2 in, 2 out]
              }
            }
            n197 = Initialize Array(w384) -> (w387:T7[])  [unwired: 1 in]
            n198 = Number To Decimal String(number=0) -> (decimal integer string=w377:string)  [unwired: 1 in]
            n199 = Number To Decimal String(number=w345) -> (decimal integer string=w376:string)  [unwired: 1 in]
            n200 = Insert Into Array(array=w387, new element=w385) -> (w386:T7[])  [unwired: 1 in]
            n201 = Format Into String(w372) -> (resulting string=w371:string)  [unwired: 3 in, 1 out]
            n202 = call <vilib>:"Space Constant.vi"() -> ("String"=w374:string)
            n203 = Array To Spreadsheet String(delimiter (Tab)=w374, array=w369, 3:"%02X" ("format string")) -> (spreadsheet string=w367:string)
            n204 = call <instrlib>:"Write.vi"("error in"=w350, "Messages"=w386, "Number to Write"=1, "CanHandleIn"=w380) -> ("error out"=w383:errorcluster, "CanHandleOut"=w381:T5)  [unwired: 4 in]
            n205 = Initialize Array("") -> (w375:string[])  [unwired: 1 in]
            n206 = Insert Into Array(array=w375, new element #1=w371, new element #2="Tx" ("new element/subarray"), new element #3=w378, new element #4=w377, new element #5=w376, new element #6=w367) -> (w366:string[])  [unwired: 1 in]
            n207 = Insert Into Array(array=w358, new element=w366) -> (w360:string[][])  [unwired: 2 in]
            n208 = local write "Table Control"(w360) -> ()
          }
          event Key Down {
            # "Key  ScanCode\n  A        30\n  B        48\n  C        46"
            n209 = event-data() -> ("ScanCode"=w431:i16, "PlatMods"=w426:T9)  [unwired: 1 in, 7 out]
            n210 = local read "ledOpen"() -> (w423:bool)
            n211 = Unbundle By Name(w426) -> ("Shift"=w425:bool)
            n212 = Compound Arithmetic op=AND(w425, w423) -> (w424:bool)
            n213 = case shown="True" w424 {
              tunnel: w431 -> [_ w432]
              frame False {
              }
              frame True {
                n214 = case shown="46" w432 {
                  frame 0, Default {
                  }
                  frame 30 {
                    n215 = property on="buttonSendA" class="Bool (strict)"("Val(Sgnl)"=TRUE ("Value (Signaling)")) -> ()  [unwired: 2 in, 2 out]
                  }
                  frame 48 {
                    n216 = property on="buttonSendB" class="Bool (strict)"("Val(Sgnl)"=TRUE ("Value (Signaling)")) -> ()  [unwired: 2 in, 2 out]
                  }
                  frame 46 {
                    n217 = property on="buttonSendC" class="Bool (strict)"("Val(Sgnl)"=TRUE ("Value (Signaling)")) -> ()  [unwired: 2 in, 2 out]
                  }
                }
              }
            }
          }
          event "buttonPause": Value Change {
            w436 = T1."Disabled and Grayed Out" ("Disabled")
            w438 = T1."Enabled" ("Disabled")
            n218 = event-data() -> ()  [unwired: 1 in, 5 out]
            n219 = call <instrlib>:"Close.vi"("error in"=w446, "CanHandleIn"=w444) -> ("error out"=w445:errorcluster, "CanHandleOut"=w443:T5)  [unwired: 8 in]
            n220 = call <instrlib>:"Disconnect.vi"("error in"=w445, "CanHandleIn"=w443) -> ("error out"=w447:errorcluster)  [unwired: 9 in]
            n221 = property on="buttonSendA" class="Bool (strict)"("DisabledEnum"=w436) -> ()  [unwired: 2 in, 2 out]
            n222 = property on="buttonSendC" class="Bool (strict)"("DisabledEnum"=w436) -> ()  [unwired: 2 in, 2 out]
            n223 = property on="buttonSendB" class="Bool (strict)"("DisabledEnum"=w436) -> ()  [unwired: 2 in, 2 out]
            n224 = local write "Fw Revision"("" ("Firmware Revision")) -> ()
            n225 = local write "Serial Number"("" ("Serial Number")) -> ()
            n226 = local write "Asm Version"("" ("Asm Version")) -> ()
            n227 = property on="checkBoxNoAutoTx" class="Bool (strict)"("DisabledEnum"=w438) -> ()  [unwired: 2 in, 2 out]
            n228 = property on="checkBoxLoopback" class="Bool (strict)"("DisabledEnum"=w438) -> ()  [unwired: 2 in, 2 out]
            n229 = property on="checkBoxListenOnly" class="Bool (strict)"("DisabledEnum"=w438) -> ()  [unwired: 2 in, 2 out]
            n230 = property on="Tab" class="TabCtl (strict)"("DisabledEnum"=w438) -> ()  [unwired: 2 in, 2 out]
            n231 = property on="comboBaudRate" class="Ring (strict)"("DisabledEnum"=w438) -> ()  [unwired: 2 in, 2 out]
            n232 = property on="comboAdapters" class="Ring (strict)"("DisabledEnum"=w438) -> ()  [unwired: 2 in, 2 out]
            n233 = property on="buttonPlay" class="Bool"("DisabledEnum"=w438) -> ()  [unwired: 2 in, 2 out]
            n234 = local write "ledOpen"(FALSE ("IndicatorOpen")) -> ()
            n235 = property on="buttonPause" class="Bool"("DisabledEnum"=w436) -> ()  [unwired: 2 in, 2 out]
            n236 = property on="checkBoxTermination" class="Bool (strict)"("DisabledEnum"=w438) -> ()  [unwired: 2 in, 2 out]
          }
        }
        "ledStop" <- w76
        n237 = case shown="No Error" w78 {
          selector: w78 -> [w87 w91]
          tunnel: [w87 w93] -> w75
          tunnel: [FALSE w92] -> w77
          frame No Error {
          }
          frame Error {
            n238 = call <vilib>:"Simple Error Handler.vi"("error in (no error)"=w91) -> ("error out"=w89:errorcluster)  [unwired: 4 in, 4 out]
            n239 = flat-sequence {
              tunnel: [w98] -> w90
              tunnel: w89 -> [w98]
              tunnel: [w94] -> w88
              frame #0 {
                n240 = Two Button Dialog(message="Stop or Continue", 1:"Stop App" ("T button name (\"OK\")"), 2:"Continue" ("message")) -> (T button?=w94:bool)
              }
            }
            n241 = case shown="True" w88 {
              tunnel: [w99 w101] -> w93
              tunnel: w90 -> [w99 w100]
              frame False {
              }
              frame True {
                n242 = call <vilib>:"Clear Errors.vi"("error in (no error)"=w100) -> ("error out"=w101:errorcluster)  [unwired: 6 in]
              }
            }
            n243 = Not(x=w88) -> (.not. x?=w92:bool)
          }
        }
        n244 = Or(x=w77, y=w76) -> (x .or. y?=w79:bool)
      }
    }
    frame Error {
    }
  }
  n245 = call <instrlib>:"Disconnect.vi"("error in"=w19, "CanHandleIn"=w54) -> ("error out"=w36:errorcluster)  [unwired: 9 in]
  n246 = disable-structure shown="RUN_TIME_ENGINE==True" {
    disable-tunnel: w36 -> [w451 w453]
    disable-tunnel: [w451 w452] -> _
    frame condition #0 (active) {
    }
    frame condition #1 {
      n247 = control-ref of="This VI"() -> (w455:refnum<vi>)
      n248 = invoke class="VI" method="FP.Close"(reference=w455, error in=w453) -> (reference out=w454:refnum<vi>, error out=w456:errorcluster)  [unwired: 1 in, 1 out]
      n249 = Close Reference(reference=w454, error in (no error)=w456) -> (error out=w452:errorcluster)
    }
  }
